vi "Query PCB Temperature.vi"(8 "error in (no error)":errorcluster, 11 "VISA resource name":refnum<visa-resource-name>) -> (0 "error out":errorcluster, 2 "PCB Temperature":dbl, 3 "VISA resource name out":refnum<visa-resource-name>)   [LabVIEW 2021, in "Ocean Optics 2000 4000.lvlib"]
doc: "Returns the instrument's printed circuit board(PCB) temperature."
uses:
  <instrlib>/Ocean Optics 2000 4000/Ocean Optics 2000 4000.lvlib
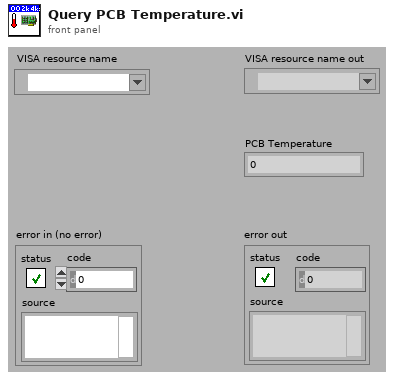
[diagram p1: front panel]
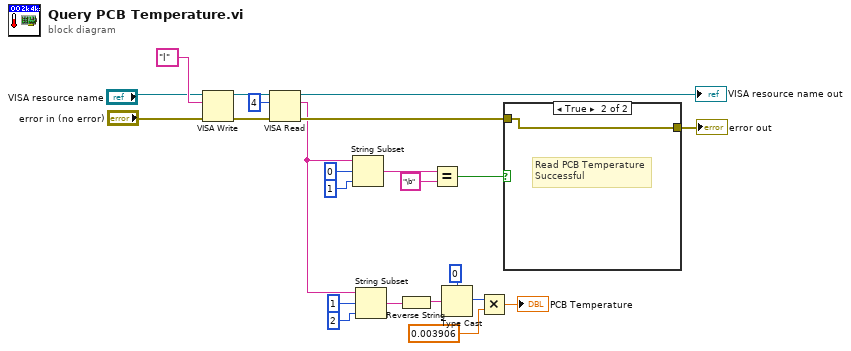
[diagram p0: block diagram]
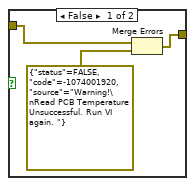
[diagram p2: hidden frame]
diagram:
  n1 = VISA Write(VISA resource name="VISA resource name", write buffer="l", error in (no error)="error in (no error)") -> (VISA resource name out=w21:refnum<visa-resource-name>, error out=w22:errorcluster)  [unwired: 1 out]
  n2 = VISA Read(VISA resource name=w21, byte count=u32 4, error in (no error)=w22) -> (VISA resource name out=→"VISA resource name out":refnum<visa-resource-name>, read buffer=w7:string, error out=w11:errorcluster)  [unwired: 1 out]
  n3 = String Subset(string=w7, offset (0)=0, length (rest)=1 ("length (rest)")) -> (substring=w14:string)
  n4 = String Subset(string=w7, offset (0)=1, length (rest)=2 ("length (rest)")) -> (substring=w6:string)
  n5 = Reverse String(1:w6) -> (0:w5:string)
  n6 = Equal?(x=w14, y="\b") -> (x = y?=w12:bool)
  n7 = Type Cast(type=u16 0, x=w5) -> (*(type *) &x=w3:u16)
  n8 = Multiply(x=w3, y=0.003906) -> (x*y=→"PCB Temperature":dbl)
  n9 = case shown="True" w12 {
    tunnel: w11 -> [w26 w27]
    tunnel: [w24 w27] -> w10
    frame False {
      n10 = Merge Errors(w26, errorcluster {"status"=FALSE, "code"=-1074001920, "source"="Warning!\nRead PCB Temperature Unsuccessful. Run VI again. "} ("error in 2 (no error)")) -> (w24:errorcluster)
    }
    frame True {
      # "Read PCB Temperature Successful"
    }
  }
  "error out" <- w10
